vi "Open.vi"(8 "error in (no error)":errorcluster, 9 "waitForOpenDone(ms)":i32, 10 "exe path":path, 11 "LT_UpgradeFlash in":refnum<class "LT_UpgradeFlash.lvclass">) -> (0 "error out":errorcluster, 1 "resultStr":string, 2 "ActionResult":bool, 3 "LT_UpgradeFlash out":refnum<class "LT_UpgradeFlash.lvclass">)   [LabVIEW 2017, in "LT_UpgradeFlash.lvclass"]
uses:
  LT_UpgradeFlash.lvclass
  D:/Project/Tymphany/LT_UpgradeFlash/New_Lib/LT_UpgradeFlash_dll/LT_UpgradeFlash_dll/bin/Debug/LT_UpgradeFlash_dll.dll
  New_Lib/LT_UpgradeFlash_dll/LT_UpgradeFlash_dll/bin/Debug/LT_UpgradeFlash_dll.dll
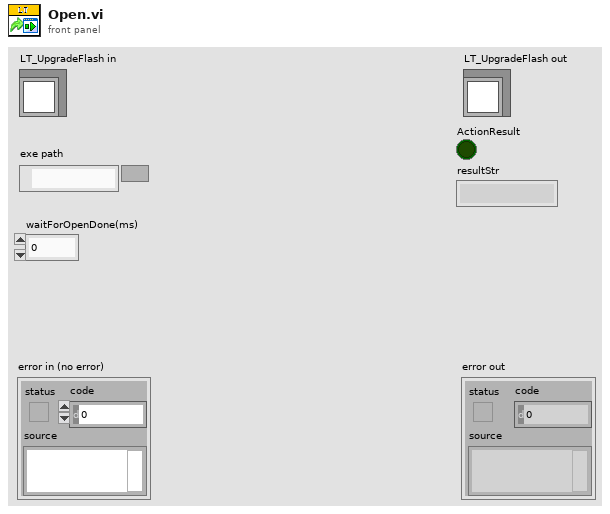
[diagram p1: front panel]
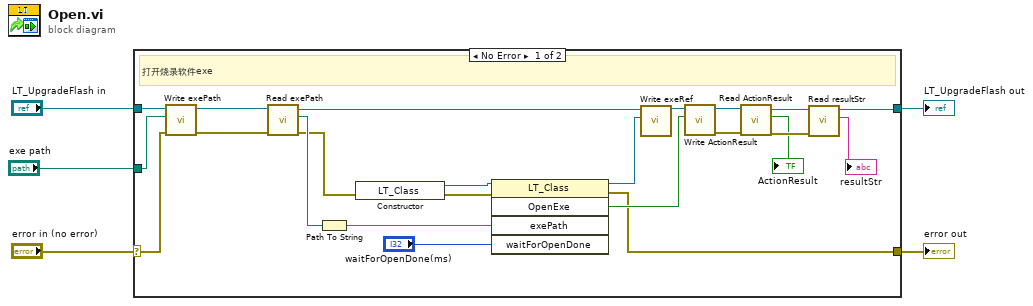
[diagram p0: block diagram]
diagram:
  n1 = case shown="No Error" "error in (no error)" {
    selector: "error in (no error)" -> [w18 w30]
    tunnel: [w22 w30] -> w4
    tunnel: [w11 w29] -> w2
    tunnel: "LT_UpgradeFlash in" -> [w21 w29]
    tunnel: "exe path" -> [w16 _]
    frame No Error {
      # "打开烧录软件exe"
      n2 = call-dynamic "Write exePath.vi"("error in (no error)"=w18, "exePath"=w16, "LT_UpgradeFlash in"=w21) -> ("error out"=w19:errorcluster, "LT_UpgradeFlash out"=w20:refnum<class "LT_UpgradeFlash.lvclass">)  [unwired: 7 in]
      n3 = call-dynamic "Read exePath.vi"("error in (no error)"=w19, "LT_UpgradeFlash in"=w20) -> ("error out"=w17:errorcluster, "exePath"=w28:path, "LT_UpgradeFlash out"=w25:refnum<class "LT_UpgradeFlash.lvclass">)  [unwired: 7 in]
      n4 = Path To String(path=w28) -> (string=w27:string)
      n5 = constructor class="LT_Class"(error in=w17) -> (reference out=w8:refnum<k24>, error out=w23:errorcluster)  [unwired: 2 in, 1 out]
      n6 = invoke class="LT_Class" method="OpenExe"(reference=w8, error in=w23, "exePath"=w27, "waitForOpenDone"="waitForOpenDone(ms)") -> (reference out=w7:refnum<k24>, error out=w22:errorcluster, "OpenExe"=w26:bool)  [unwired: 1 in, 2 out]
      n7 = call-dynamic "Write exeRef.vi"("exeRef"=w7, "LT_UpgradeFlash in"=w25) -> ("LT_UpgradeFlash out"=w24:refnum<class "LT_UpgradeFlash.lvclass">)  [unwired: 8 in, 1 out]
      n8 = call-dynamic "Write ActionResult.vi"("ActionResult"=w26, "LT_UpgradeFlash in"=w24) -> ("error out"=w14:errorcluster, "LT_UpgradeFlash out"=w15:refnum<class "LT_UpgradeFlash.lvclass">)  [unwired: 8 in]
      n9 = call-dynamic "Read ActionResult.vi"("error in (no error)"=w14, "LT_UpgradeFlash in"=w15) -> ("error out"=w12:errorcluster, "ActionResult"=→"ActionResult":bool, "LT_UpgradeFlash out"=w13:refnum<class "LT_UpgradeFlash.lvclass">)  [unwired: 7 in]
      n10 = call-dynamic "Read resultStr.vi"("error in (no error)"=w12, "LT_UpgradeFlash in"=w13) -> ("resultStr"=→"resultStr":string, "LT_UpgradeFlash out"=w11:refnum<class "LT_UpgradeFlash.lvclass">)  [unwired: 7 in, 1 out]
    }
    frame Error {
    }
  }
  "error out" <- w4
  "LT_UpgradeFlash out" <- w2
